vi "Simple vi.vi"() -> ()   [LabVIEW 2014]
uses:
  <vilib>/Utility/error.llb/DialogType.ctl
panel:
  in  "stop":bool
  out "error out":errorcluster
  out "out":dbl
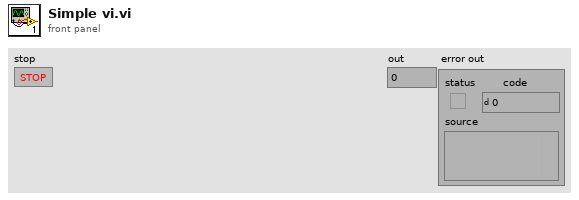
[diagram p1: front panel]
types:
  T1 = typedef "DialogType.ctl" = u16
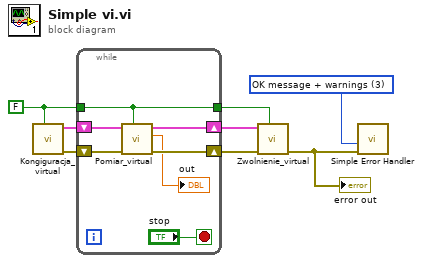
[diagram p0: block diagram]
diagram:
  w3 = T1 3 items=["no dialog", "OK message", "continue or stop message", "OK message + warnings", "continue/stop + warnings"] ("type of dialog (OK msg:1)")
  w1 = FALSE ("Error Generate")
  n1 = call "Kongiguracja_virtual.vi"("Error Generate"=w1) -> ("error out"=w7:errorcluster, "Reference out"=w8:cluster{"Numeric":dbl, "Boolean":bool})  [unwired: 9 in]
  n2 = while {
    tunnel: w1 -> [w11]
    shift-right: [w12] -> w5
    shift-left: w8 -> [w15]
    shift-right: [w13] -> w6
    shift-left: w7 -> [w14]
    tunnel: [w11] -> w2
    stop <- "stop" stop-if-true
    n3 = call "Pomiar_virtual.vi"("Error Generate"=w11, "error in (no error)"=w14, "Reference in"=w15) -> ("error out"=w13:errorcluster, "out"=→"out":dbl, "Reference out"=w12:cluster{"Numeric":dbl, "Boolean":bool})  [unwired: 6 in]
  }
  n4 = call "Zwolnienie_virtual.vi"("Error Generate"=w2, "error in (no error)"=w6, "Reference in"=w5) -> ("error out"=w4:errorcluster)  [unwired: 8 in]
  "error out" <- w4
  n5 = call <vilib>:"Simple Error Handler.vi"("type of dialog (OK msg:1)"=w3, "error in (no error)"=w4) -> ()  [unwired: 3 in, 5 out]
